vi "lv9_model_Core_1.vi"() -> ()   [LabVIEW 2009]
doc: "This example demonstrates how to continuously acquire buffered voltage measurements using a DAQmx device.\n\nFor instructions on how to connect your signals to the DAQ device, refer to your device documentation."
uses:
  <libdir>/resource/objmgr/daqmx.rc
  <vilib>/DAQmx/read.llb/DAQmx Read (Analog 1D Wfm NChan NSamp).vi
  <vilib>/DAQmx/create/channels.llb/DAQmx Create Channel (AI-Voltage-Basic).vi
  <vilib>/DAQmx/configure/timing.llb/DAQmx Timing (Sample Clock).vi
panel:
  in  "Stop":bool
  out "Waveform Graph":waveform(dbl)[](graph)
  in  "Samples per Loop":i32
  in  "Sample Rate":dbl
  in  "Sample Clock Source":tag
  in  "Terminal Configuration":i32(ring) items=["default", "RSE", "NRSE", "Differential", "Pseudodifferential"]
  in  "Max Voltage":dbl
  in  "Min Voltage":dbl
  in  "Physical Channel":tag
  out "Actual Sample Rate":dbl format="%0.2f"
  # "Channel Settings"
  # "Trigger Settings"
  # "Acquired Data"
  # "Timing Settings"
  # "Logging Settings"
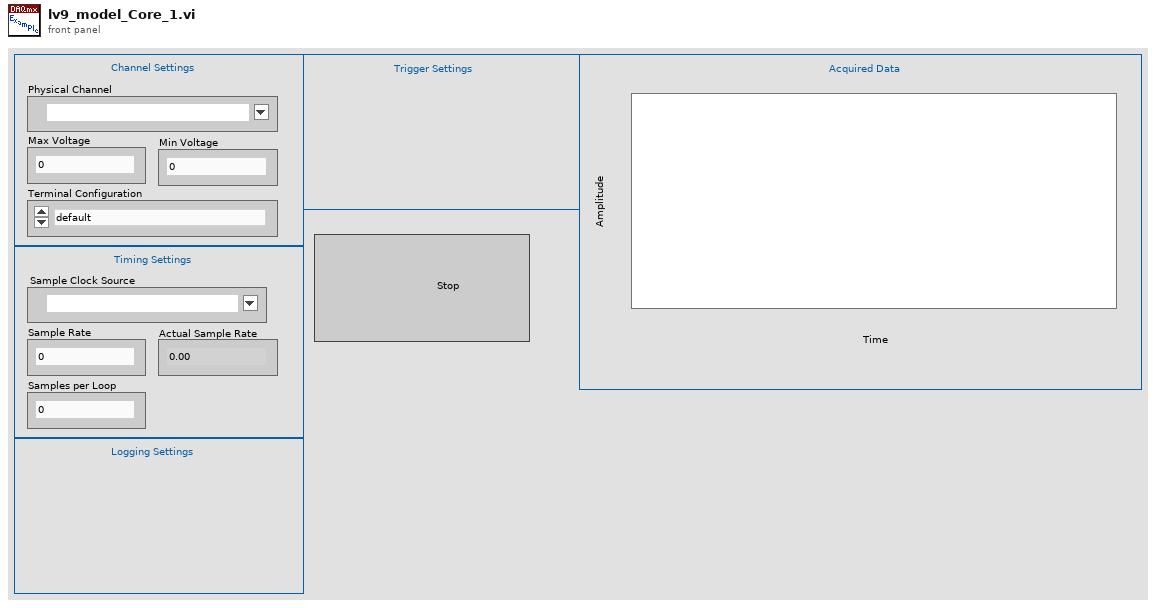
[diagram p1: front panel]
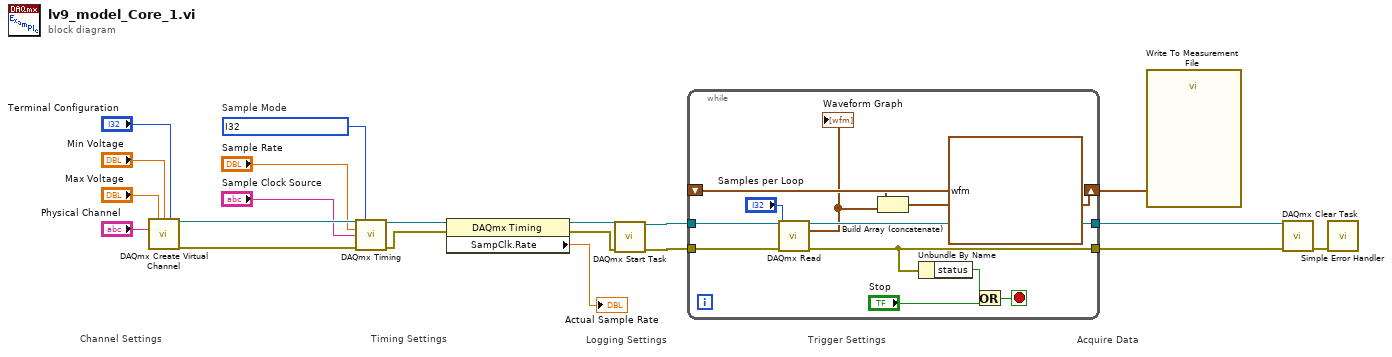
[diagram p0: block diagram]
diagram:
  w19 = i32 ? items=["Finite Samples", "Continuous Samples", "Hardware Timed Single Point"]  # Sample Mode
  # "Trigger Settings"
  # "Acquire Data"
  # "Timing Settings"
  # "Channel Settings"
  # "Logging Settings"
  n1 = call-poly <vilib>:"DAQmx Create Virtual Channel.vi"("maximum value"="Max Voltage", "minimum value"="Min Voltage", "input terminal configuration"="Terminal Configuration", "physical channels"="Physical Channel") -> ("task out"=w17:refnum<k21>, "error out"=w18:errorcluster)  [unwired: 10 in]
  n2 = call-poly <vilib>:"DAQmx Timing.vi"("task/channels in"=w17, "sample mode"=w19, "rate"="Sample Rate", "source"="Sample Clock Source", "error in"=w18) -> ("task out"=w21:refnum<k21>, "error out"=w20:errorcluster)  [unwired: 9 in]
  n3 = property class="DAQmx Timing"(reference=w21, error in=w20) -> (reference out=w4:refnum<k21>, error out=w3:errorcluster, "SampClk.Rate"=→"Actual Sample Rate":dbl)
  n4 = call <vilib>:"DAQmx Start Task.vi"("task/channels in"=w4, "error in"=w3) -> ("task out"=w16:refnum<k21>, "error out"=w15:errorcluster)  [unwired: 12 in]
  n5 = while {
    tunnel: w16 -> [w32]
    tunnel: w15 -> [w31]
    tunnel: [w29] -> w13
    tunnel: [w25] -> w14
    shift-right: [w22] -> w2
    shift-left: waveform(dbl)[] ? ("data") -> [w23]
    stop <- w30 stop-if-true
    n6 = call-poly <vilib>:"DAQmx Read.vi"("task/channels in"=w32, "number of samples per channel"="Samples per Loop", "error in"=w31) -> ("task out"=w25:refnum<k21>, "data"=w24:waveform(dbl)[], "error out"=w29:errorcluster)  [unwired: 10 in]
    "Waveform Graph" <- w24
    n7 = Build Array (concatenate)(w23, w24) -> (w22:waveform(dbl)[])
    n8 = Unbundle By Name(w29) -> ("status"=w28:bool)
    n9 = Or(x=w28, y="Stop") -> (x .or. y?=w30:bool)
  }
  n10 = call "Write To Measurement File"("Signals"=w2) -> ()  [unwired: 16 in, 3 out]
  n11 = call <vilib>:"DAQmx Clear Task.vi"("task in"=w14, "error in"=w13) -> ("error out"=w12:errorcluster)  [unwired: 13 in]
  n12 = call <vilib>:"Simple Error Handler.vi"("error in (no error)"=w12) -> ()  [unwired: 4 in, 5 out]
